vi "Read Ramp Rate.vi"(11 "PressureValve in":refnum<class "PressureValve.lvclass">) -> (2 "Ramp Rate":dbl[unit]=2.0 min=0.001 max=4.0 format="%.3f", 3 "PressureValve out":refnum<class "PressureValve.lvclass">)   [LabVIEW 2015]
uses:
  <userlib>/Common/Devices/PressureValve/PressureValve/PressureValve.lvclass
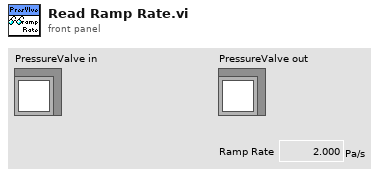
[diagram p1: front panel]
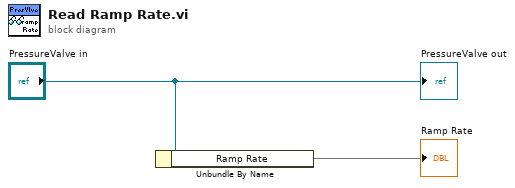
[diagram p0: block diagram]
diagram:
  n1 = Unbundle By Name("PressureValve in") -> ("Ramp Rate"=→"Ramp Rate")
  "PressureValve out" <- "PressureValve in"
